vi "Respuestas.vi"() -> ()   [LabVIEW 2016]
panel:
  out "Respuesta":string
  in  "Entrada":string
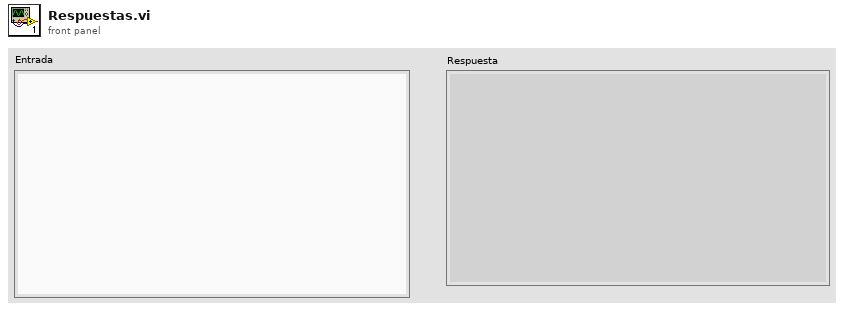
[diagram p1: front panel]
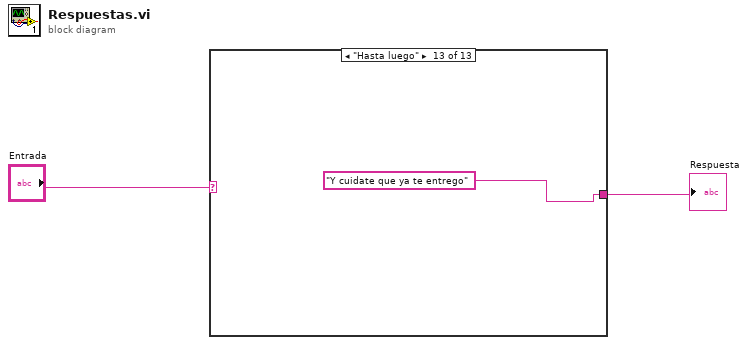
[diagram p0: block diagram]
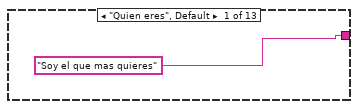
[diagram p2: hidden frame]
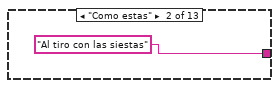
[diagram p3: hidden frame]
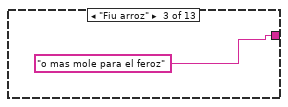
[diagram p4: hidden frame]
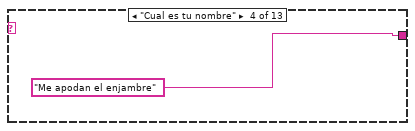
[diagram p5: hidden frame]
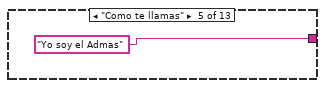
[diagram p6: hidden frame]
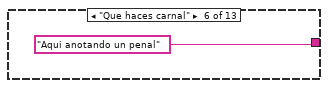
[diagram p7: hidden frame]
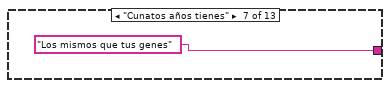
[diagram p8: hidden frame]
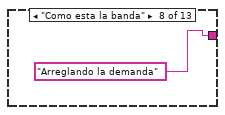
[diagram p9: hidden frame]
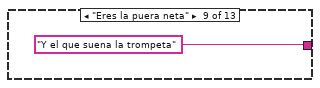
[diagram p10: hidden frame]
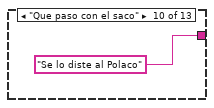
[diagram p11: hidden frame]
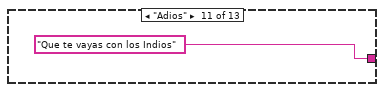
[diagram p12: hidden frame]
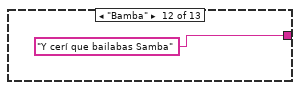
[diagram p13: hidden frame]
diagram:
  n1 = case shown="\"Hasta luego\"" "Entrada" {
    tunnel: ["Soy el que mas quieres" "Al tiro con las siestas" "o mas mole para el feroz" "Me apodan el enjambre" "Yo soy el Admas" "Aqui anotando un penal" "Los mismos que tus genes" "Arreglando la demanda" "Y el que suena la trompeta" "Se lo diste al Polaco" "Que te vayas con los Indios" "Y cerí que bailabas Samba" "Y cuidate que ya te entrego"] -> w1
    frame "Quien eres", Default {
    }
    frame "Como estas" {
    }
    frame "Fiu arroz" {
    }
    frame "Cual es tu nombre" {
    }
    frame "Como te llamas" {
    }
    frame "Que haces carnal" {
    }
    frame "Cunatos años tienes" {
    }
    frame "Como esta la banda" {
    }
    frame "Eres la puera neta" {
    }
    frame "Que paso con el saco" {
    }
    frame "Adios" {
    }
    frame "Bamba" {
    }
    frame "Hasta luego" {
    }
  }
  "Respuesta" <- w1
